vi "ORS_GalvoCleanupScan.vi"(8 "error in":errorcluster, 10 "cleanupgalvo":bool, 11 "Galvo":T1={"x mirror"="", "y mirror"="", "trig out"="", "x mirror task"="", "y mirror task"="", "trig out task"="", "n_axis"=0, "params"={"n_lines"=512, "n_frames"=1, "force to zero"=FALSE, "Triggers_per_sweep"=0.0, "X center"=0.0, "X span"=0.0, "Y center"=0.0, "Y span"=0.0, "flyb.lines"=0, "n_triggers"=0, "mode"=0, "offset"=5.0, "galvo phase"=0, "span factor"=1.0, "Custom trig."={"n_f to c. trig"=150, "c. trig length"=8, "c. trig interval"=1024, "n_c. trig"=1}, "f_per_pos"=1, "n_dataset"=1, "flyback fr"=1}, "acq trig out"="", "acq trig out task"="", "sample array X"=[], "sample array Y"=[], "custom trig out"="Dev1/port0/line7", "custom trig out task"="", "FDML-box"="TCPIP0::10.153.218.51::23::SOCKET", "ACQ/Galvo"=enum."ADC/FDML", "acq trig out an task"="", "acq trig out an"="", "Galvo Trig input"="", "Galvo Clk input"="", "sample array Acq trig out an"=[]} {"params"."n_dataset" min=1; "params"."X center" format="%^_3g"; "params"."X span" format="%^_3g"; "params"."Y center" format="%^_3g"; "params"."Y span" format="%^_3g"}) -> (0 "error out":errorcluster, 3 "Galvo out":T1={"x mirror"="", "y mirror"="", "trig out"="", "x mirror task"="", "y mirror task"="", "trig out task"="", "n_axis"=0, "params"={"n_lines"=512, "n_frames"=1, "force to zero"=FALSE, "Triggers_per_sweep"=0.0, "X center"=0.0, "X span"=0.0, "Y center"=0.0, "Y span"=0.0, "flyb.lines"=0, "n_triggers"=0, "mode"=0, "offset"=5.0, "galvo phase"=0, "span factor"=1.0, "Custom trig."={"n_f to c. trig"=150, "c. trig length"=8, "c. trig interval"=1024, "n_c. trig"=1}, "f_per_pos"=1, "n_dataset"=1, "flyback fr"=1}, "acq trig out"="", "acq trig out task"="", "sample array X"=[], "sample array Y"=[], "custom trig out"="Dev1/port0/line7", "custom trig out task"="", "FDML-box"="TCPIP0::10.153.218.51::23::SOCKET", "ACQ/Galvo"=enum."ADC/FDML", "acq trig out an task"="", "acq trig out an"="", "Galvo Trig input"="", "Galvo Clk input"="", "sample array Acq trig out an"=[]} {"params"."n_dataset" min=1; "params"."X center" format="%^_3g"; "params"."X span" format="%^_3g"; "params"."Y center" format="%^_3g"; "params"."Y span" format="%^_3g"})   [LabVIEW 2021]
uses:
  Typedefs/ORS_Galvo.ctl
  Typedefs/ORS_Galvo_params.ctl
  <vilib>/Utility/error.llb/DialogType.ctl
  <vilib>/DAQmx/write.llb/DAQmx Write (Analog 1D DBL NChan 1Samp).vi
  <vilib>/DAQmx/miscellaneous.llb/DAQmx Fill In Error Info.vi
  <resource>/objmgr/daqmx.rc
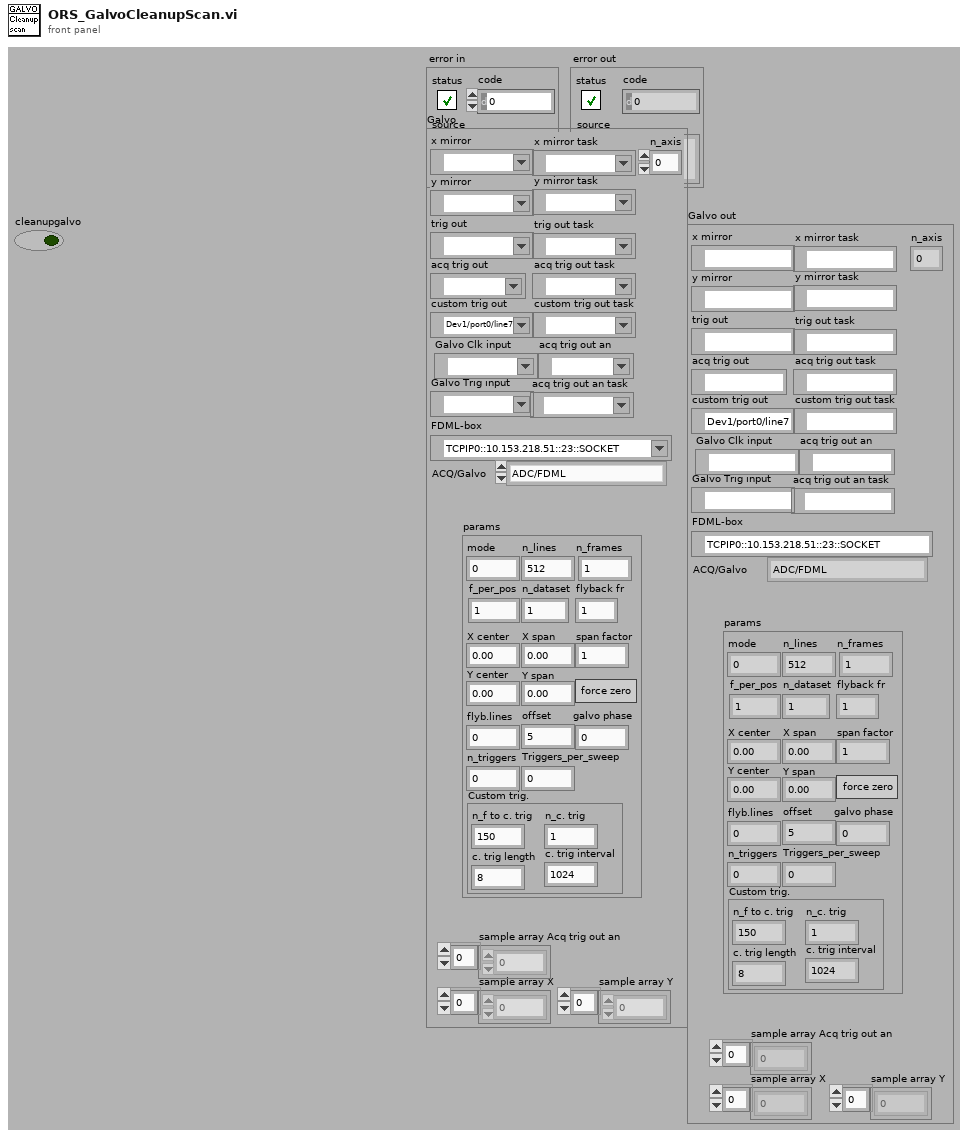
[diagram p1: front panel]
types:
  T1 = typedef "ORS_Galvo.ctl" = cluster{"x mirror":tag, "y mirror":tag, "trig out":tag, "x mirror task":refnum<k21>, "y mirror task":refnum<k21>, "trig out task":refnum<k21>, "n_axis":i32, "params":T2, "acq trig out":tag, "acq trig out task":refnum<k21>, "sample array X":dbl[], "sample array Y":dbl[], "custom trig out":tag, "custom trig out task":refnum<k21>, "FDML-box":refnum<visa-resource-name>, "ACQ/Galvo":enum16{"ADC/FDML", "NI_DAQ", "ADC"}, "acq trig out an task":refnum<k21>, "acq trig out an":tag, "Galvo Trig input":tag, "Galvo Clk input":tag, "sample array Acq trig out an":dbl[]}
  T2 = typedef "ORS_Galvo_params.ctl" = cluster{"n_lines":i32, "n_frames":i32, "force to zero":bool, "Triggers_per_sweep":dbl, "X center":dbl, "X span":dbl, "Y center":dbl, "Y span":dbl, "flyb.lines":i32, "n_triggers":i32, "mode":i32, "offset":dbl, "galvo phase":i32, "span factor":dbl, "Custom trig.":cluster{"n_f to c. trig":i32, "c. trig length":i32, "c. trig interval":i32, "n_c. trig":i32}, "f_per_pos":i32, "n_dataset":u32, "flyback fr":u16}
  T3 = typedef "DialogType.ctl" = u16
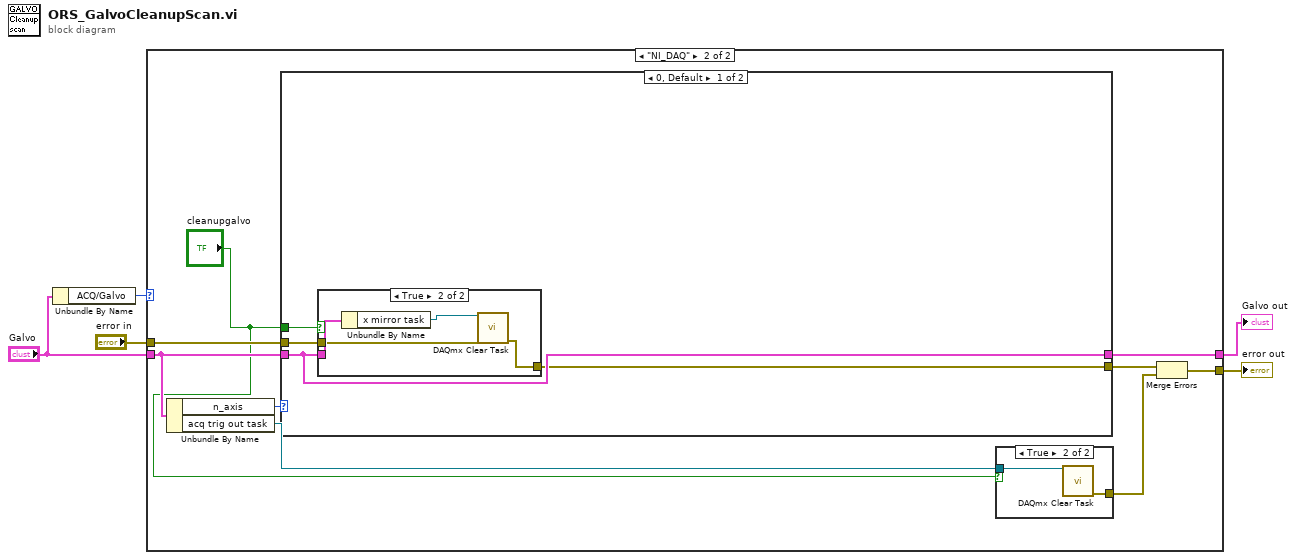
[diagram p0: block diagram]
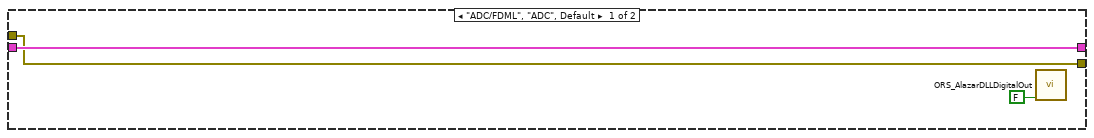
[diagram p2: hidden frame]
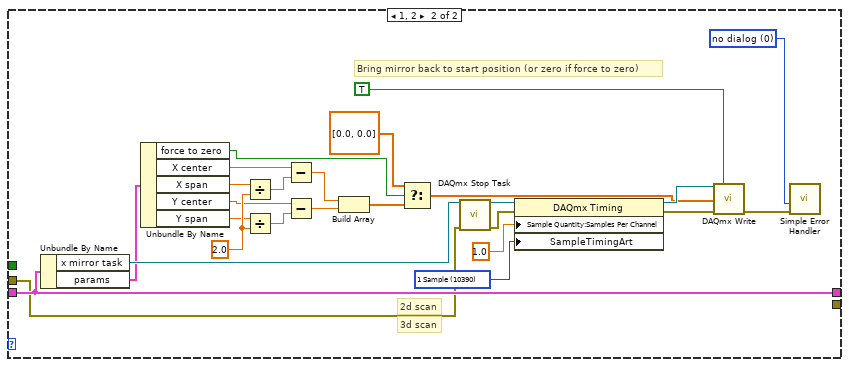
[diagram p5: hidden frame]
diagram:
  n1 = Unbundle By Name("Galvo") -> ("ACQ/Galvo"=w1:enum16{"ADC/FDML", "NI_DAQ", "ADC"})
  n2 = case shown="\"NI_DAQ\"" w1 {
    tunnel: "error in" -> [w7 w16]
    tunnel: [w7 w15] -> w4
    tunnel: "Galvo" -> [w8 w12]
    tunnel: [w8 w11] -> w3
    frame "ADC/FDML", "ADC", Default {
      n3 = call "ORS_AlazarDLLDigitalOut.vi"("level"=FALSE) -> ()  [unwired: 8 in, 3 out]
    }
    frame "NI_DAQ" {
      n4 = Unbundle By Name(w12) -> ("n_axis"=w17:i32, "acq trig out task"=w10:refnum<k21>)
      n5 = case shown="0, Default" w17 {
        tunnel: w16 -> [w22 w47]
        tunnel: [w21 _] -> w14
        tunnel: [w23 w54] -> w11
        tunnel: w12 -> [w23 w54]
        tunnel: "cleanupgalvo" -> [w20 _]
        frame 0, Default {
          n6 = case shown="True" w20 {
            tunnel: w23 -> [_ w28]
            tunnel: w22 -> [w24 w26]
            tunnel: [w24 w25] -> w21
            frame False {
            }
            frame True {
              n7 = Unbundle By Name(w28) -> ("x mirror task"=w27:refnum<k21>)
              n8 = call <vilib>:"DAQmx Clear Task.vi"("task in"=w27, "error in"=w26) -> ("error out"=w25:errorcluster)  [unwired: 13 in]
            }
          }
        }
        frame 1, 2 {
          w29 = T3 0 items=["no dialog", "OK message", "continue or stop message", "OK message + warnings", "continue/stop + warnings"] ("type of dialog (OK msg:1)")
          w44 = 2.0
          w49 = 10390 items=["Sample-Takt"=10388, "Burst-Handshake"=12548, "Handshake"=10389, "implizit"=10451, "1 Sample"=10390, "Änderungserkennung"=12504, "Sample-Takt in Pipeline"=14668] ("SampleTimingArt")
          # "2d scan"
          # "Bring mirror back to start position (or zero if force to zero)"
          # "3d scan"
          n9 = Unbundle By Name(w54) -> ("x mirror task"=w48:refnum<k21>, "params"=w33:T2)
          n10 = Unbundle By Name(w33) -> ("force to zero"=w42:bool, "X center"=w34:dbl, "X span"=w41:dbl, "Y center"=w35:dbl, "Y span"=w38:dbl)
          n11 = Divide(x=w41, y=w44) -> (x/y=w40:dbl)
          n12 = Divide(x=w38, y=w44) -> (x/y=w39:dbl)
          n13 = Subtract(x=w34, y=w40) -> (x-y=w36:dbl)
          n14 = Subtract(x=w35, y=w39) -> (x-y=w37:dbl)
          n15 = Build Array(w36, w37) -> (w31:dbl[])
          n16 = Select(t=dbl[] [0.0, 0.0] ("s? t:f"), s=w42, f=w31) -> (s? t:f=w32:dbl[])
          n17 = call <vilib>:"DAQmx Stop Task.vi"("task/channels in"=w48, "error in"=w47) -> ("task out"=w52:refnum<k21>, "error out"=w46:errorcluster)  [unwired: 12 in]
          n18 = property class="DAQmx Timing"(reference=w52, error in=w46, "Sample Quantity:Samples Per Channel"=1.0 ("SampleAnzahl.SampProKanal"), "SampleTimingArt"=w49) -> (reference out=w51:refnum<k21>, error out=w45:errorcluster)
          n19 = call-poly <vilib>:"DAQmx Write.vi"("task/channels in"=w51, "auto start"=TRUE, "data"=w32, "error in"=w45) -> ("error out"=w30:errorcluster)  [unwired: 9 in, 2 out]
          n20 = call <vilib>:"Simple Error Handler.vi"("type of dialog (OK msg:1)"=w29, "error in (no error)"=w30) -> ()  [unwired: 3 in, 5 out]
        }
      }
      n21 = case shown="True" "cleanupgalvo" {
        tunnel: [_ w19] -> w13
        tunnel: w10 -> [_ w18]
        frame False {
        }
        frame True {
          n22 = call <vilib>:"DAQmx Clear Task.vi"("task in"=w18) -> ("error out"=w19:errorcluster)  [unwired: 14 in]
        }
      }
      n23 = Merge Errors(w14, w13) -> (w15:errorcluster)
    }
  }
  "error out" <- w4
  "Galvo out" <- w3
